vi "Embdata_Creator_From_File.vi"(8 "error in (no error)":errorcluster, 9 "root path":path=path "C:/Dongfeng/Pattern_Creator_230525/ebd", 10 "Post File":string="dataSource_Post_Side.txt", 11 "Pre File":string="dataSource_Pre_Side.txt") -> (0 "error out":errorcluster, 1 "EBD Config":T1={"Lines of Pre-EBD Data"=1, "Lines of Post-EBD Data"=22, "Total EBD Block Size"=66309, "Pre-EBD Block Offset "=0, "Post-EBD Block Offset "=0}, 2 "Post-EBD Data (U8)":u8[](array[numeric]), 3 "Pre-EBD Data (U8)":u8[](array[numeric]))   [LabVIEW 2020]
uses:
  ctl/Image_EBD_Config.ctl
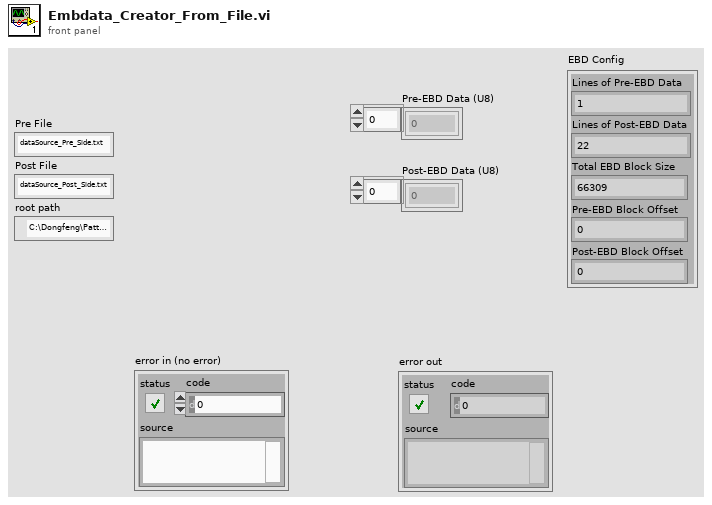
[diagram p1: front panel]
types:
  T1 = typedef "Image_EBD_Config.ctl" = cluster{"Lines of Pre-EBD Data":u16, "Lines of Post-EBD Data":u16, "Total EBD Block Size":u32, "Pre-EBD Block Offset ":u32, "Post-EBD Block Offset ":u32}
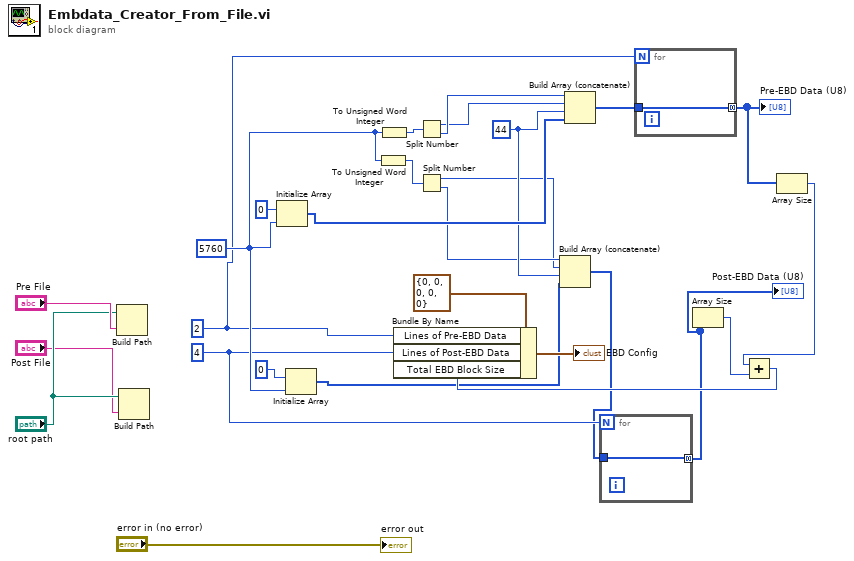
[diagram p0: block diagram]
diagram:
  w16 = u8 44 ("element")
  w15 = 5760 ("dimension size")
  w10 = u16 4 ("Lines of Post-EBD Data")
  w11 = u16 2 ("Lines of Pre-EBD Data")
  n1 = Build Path(base path="root path", name or relative path="Pre File") -> ()  [unwired: 1 out]
  n2 = Build Path(base path="root path", name or relative path="Post File") -> ()  [unwired: 1 out]
  n3 = Initialize Array(u8 0 ("element"), w15) -> (w19:u8[])
  n4 = Initialize Array(u8 0 ("element"), w15) -> (w7:u8[])
  n5 = To Unsigned Word Integer(number=w15) -> (unsigned 16bit integer=w17:u16)
  n6 = To Unsigned Word Integer(number=w15) -> (unsigned 16bit integer=w18:u16)
  n7 = Split Number(x=w18) -> (hi(x)=w3:u8, lo(x)=w4:u8)
  n8 = Split Number(x=w17) -> (hi(x)=w1:u8, lo(x)=w2:u8)
  n9 = Build Array (concatenate)(w2, w1, w16, w7) -> (w6:u8[])
  n10 = Build Array (concatenate)(w4, w3, w16, w19) -> (w9:u8[])
  n11 = for {
    N: w10 -> [_]
    tunnel: w6 -> [w28]
    tunnel: [w28] -> w5 mode=concatenating
  }
  "Post-EBD Data (U8)" <- w5
  n12 = for {
    N: w11 -> [_]
    tunnel: w9 -> [w29]
    tunnel: [w29] -> w8 mode=concatenating
  }
  "Pre-EBD Data (U8)" <- w8
  n13 = Array Size(array=w5) -> (size(s)=w13:i32)
  n14 = Array Size(array=w8) -> (size(s)=w14:i32)
  n15 = Add(x=w14, y=w13) -> (x+y=w12:i32)
  n16 = Bundle By Name(cluster=T1 {"Lines of Pre-EBD Data"=0, "Lines of Post-EBD Data"=0, "Total EBD Block Size"=0, "Pre-EBD Block Offset "=0, "Post-EBD Block Offset "=0} ("EBD Config"), "Lines of Pre-EBD Data"=w11, "Lines of Post-EBD Data"=w10, "Total EBD Block Size"=w12) -> (→"EBD Config":T1)
  "error out" <- "error in (no error)"
